vi "expand_MM.vi"(10 "xmax":dbl[](array[numeric]), 11 "centroid":dbl[](array[numeric])) -> (3 "xe":dbl[](array[numeric]))   [LabVIEW 2015]
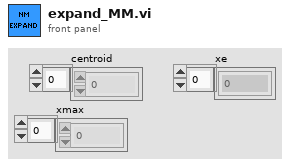
[diagram p1: front panel]
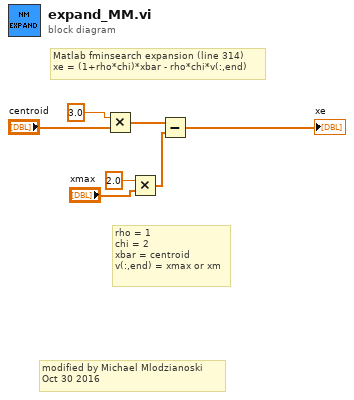
[diagram p0: block diagram]
diagram:
  # "modified by Michael Mlodzianoski\nOct 30 2016"
  # "rho = 1\nchi = 2\nxbar = centroid\nv(:,end) = xmax or xm"
  # "Matlab fminsearch expansion (line 314)\nxe = (1+rho*chi)*xbar - rho*chi*v(:,end)"
  n1 = Multiply(x=3.0, y="centroid") -> (x*y=w7:dbl[])
  n2 = Multiply(x=2.0, y="xmax") -> (x*y=w2:dbl[])
  n3 = Subtract(x=w7, y=w2) -> (x-y=→"xe":dbl[])
